vi "slop cal.vi"() -> ()   [LabVIEW 2011]
uses:
  <vilib>/Analysis/NI_AALPro.lvlib
panel:
  in  "tolerance":dbl=0.0001 format="%#_3g"
  out "slope":dbl
  out "intercept":dbl
  out "residue":dbl
  in  "x":dbl[](array[numeric])
  in  "Y":dbl[](array[numeric])
  out "XY Graph":cluster{cluster{"Numeric":dbl, dbl}[]}[](graph)
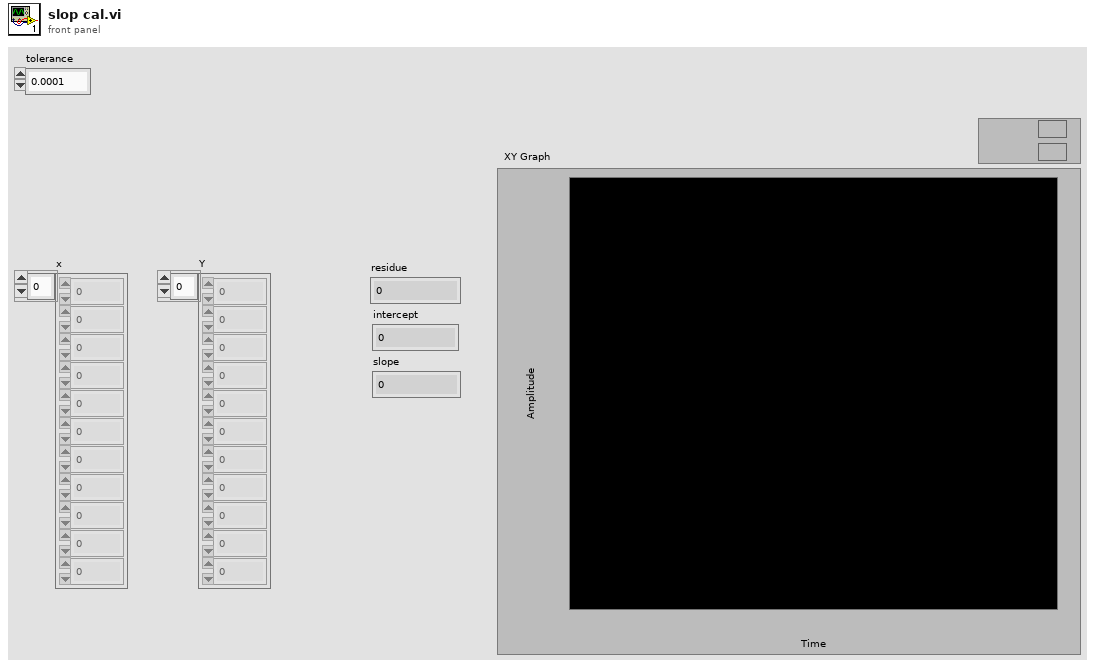
[diagram p1: front panel]
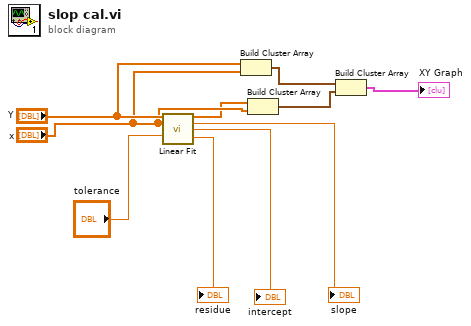
[diagram p0: block diagram]
diagram:
  n1 = call <vilib>:"Linear Fit.vi"("Y"="Y", "X"="x", "tolerance"="tolerance") -> ("Best Linear Fit"=w8:dbl[], "slope"=→"slope":dbl, "intercept"=→"intercept":dbl, "residue"=→"residue":dbl)  [unwired: 8 in, 1 out]
  n2 = Build Cluster Array ("Index & Bundle Cluster Array")("Y", "x") -> (w7:cluster{dbl, dbl}[])
  n3 = Build Cluster Array ("Index & Bundle Cluster Array")(w8, "x") -> (w6:cluster{"Numeric":dbl, dbl}[])
  n4 = Build Cluster Array(w7, w6) -> (→"XY Graph":cluster{cluster{"Numeric":dbl, dbl}[]}[])
